vi "ItemSelected.vi"(8 "error in (no error)":errorcluster, 9 "Siblings":refnum<data-value>[](array[refnum]), 10 "MenuItem in":refnum<class "MGI_MenuItem.lvclass">, 11 "SelectionType in":refnum<class "MGI_SelectionType.lvclass">) -> (0 "error out":errorcluster, 2 "MenuItem out":refnum<class "MGI_MenuItem.lvclass">, 3 "SelectionType out":refnum<class "MGI_SelectionType.lvclass">)   [LabVIEW 2016, in "MGI_SelectionType.lvclass"]
doc: "This VI will be run when the menu item is clicked.\n\nAuthored by Derek E. Trepanier\nsupport@mooregoodideas.com\nwww.mooregoodideas.com\n\nCopyright (c) 2012, Moore Good Ideas, Inc.\n\nAll rights reserved.\n\nRedistribution and use in source and binary forms, with or without modification, are permitted provided that the following conditions are met:\n\n * Redistributions of source code must retain the above copyright notice, this list of conditions and the following disclaimer.\n * Redistributions in binary form must reproduce the above copyright notice, this list of conditions and the following disclaimer in the documentation and/or other materials provided with the distribution.\n * Neither the name of Moore Good Ideas, Inc. nor the names of its contributors may be used to endorse or promote products derived from this software without specific prior written permission.\n\nTHIS SOFTWARE IS PROVIDED BY THE COPYRIGHT HOLDERS AND CONTRIBUTORS \"AS IS\" AND ANY EXPRESS OR IMPLIED WARRANTIES, INCLUDING, BUT NOT LIMITED TO, THE IMPLIED WARRANTIES OF MERCHANTABILITY AND FITNESS FOR A PARTICULAR PURPOSE ARE DISCLAIMED. IN NO EVENT SHALL THE COPYRIGHT OWNER OR CONTRIBUTORS BE LIABLE FOR ANY DIRECT, INDIRECT, INCIDENTAL, SPECIAL, EXEMPLARY, OR CONSEQUENTIAL DAMAGES (INCLUDING, BUT NOT LIMITED TO, PROCUREMENT OF SUBSTITUTE GOODS OR SERVICES; LOSS OF USE, DATA, OR PROFITS; OR BUSINESS INTERRUPTION) HOWEVER CAUSED AND ON ANY THEORY OF LIABILITY, WHETHER IN CONTRACT, STRICT LIABILITY, OR TORT (INCLUDING NEGLIGENCE OR OTHERWISE) ARISING IN ANY WAY OUT OF THE USE OF THIS SOFTWARE, EVEN IF ADVISED OF THE POSSIBILITY OF SUCH DAMAGE."
uses:
  <userlib>/_MGI/Menu Building/SelectionType/MGI_SelectionType.lvclass
  <userlib>/_MGI/Menu Building/MenuItem/MGI_MenuItem.lvclass
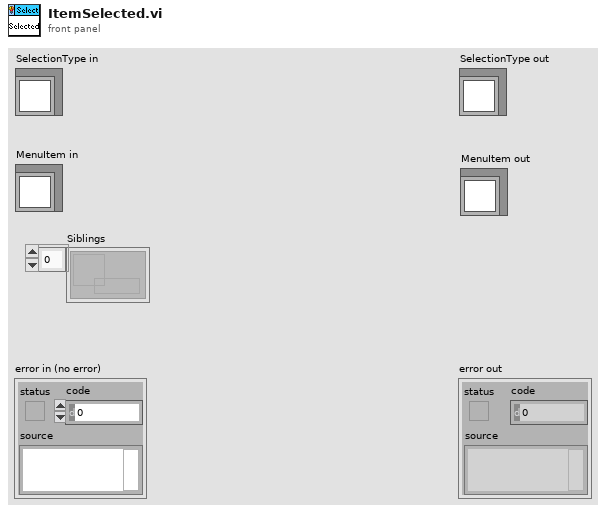
[diagram p1: front panel]
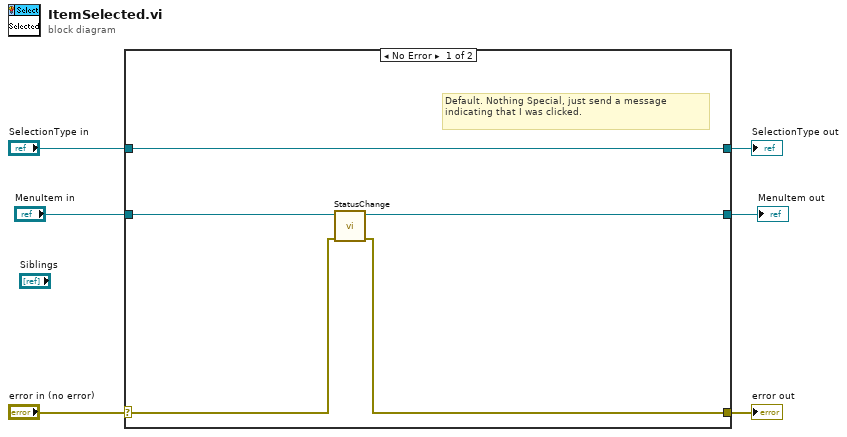
[diagram p0: block diagram]
diagram:
  n1 = case shown="No Error" "error in (no error)" {
    selector: "error in (no error)" -> [w8 w14]
    tunnel: [w10 w14] -> w5
    tunnel: [w11 w13] -> w3
    tunnel: "SelectionType in" -> [w11 w13]
    tunnel: "MenuItem in" -> [w7 w12]
    tunnel: [w9 w12] -> w1
    frame No Error {
      # "Default. Nothing Special, just send a message indicating that I was clicked."
      n2 = call-dynamic "StatusChange.vi"("error in (no error)"=w8, "MGI_MenuItem in"=w7) -> ("error out"=w10:errorcluster, "MGI_MenuItem out"=w9:refnum<class "MGI_MenuItem.lvclass">)  [unwired: 8 in]
    }
    frame Error {
    }
  }
  "error out" <- w5
  "SelectionType out" <- w3
  "MenuItem out" <- w1
